vi "Generate Header Vectors.vi"(0 "RFFE RegRead Command in":refnum<class "RFFE RegRead Command.lvclass">, 11 "error in (no error)":errorcluster) -> (4 "RFFE RegRead Command out":refnum<class "RFFE RegRead Command.lvclass">, 6 "Header Vectors":string[](array[string]), 15 "error out":errorcluster)   [LabVIEW 2018, in "MIPI RFFE API.lvlib" / "RFFE RegRead Command.lvclass"]
uses:
  RFFE RegRead Command.lvclass
  Standard Command/RFFE Standard Command.lvclass
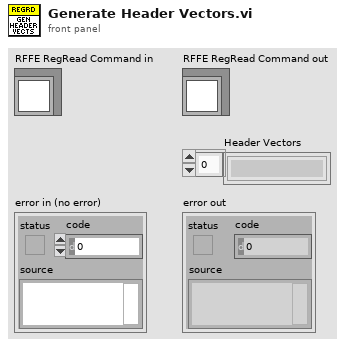
[diagram p1: front panel]
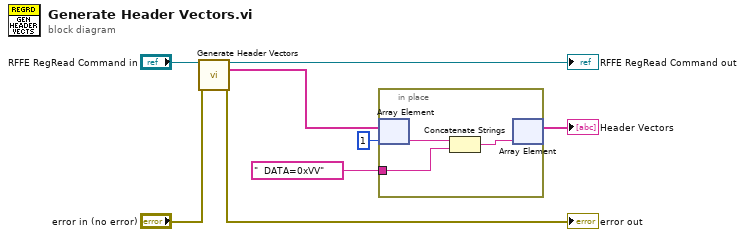
[diagram p0: block diagram]
diagram:
  n1 = call-parent "Generate Header Vectors.vi"("RFFE Command in"="RFFE RegRead Command in", "error in (no error)"="error in (no error)") -> ("RFFE Command out"=→"RFFE RegRead Command out":refnum<class "RFFE RegRead Command.lvclass">, "Header Vectors"=w3:string[], "error out"=→"error out":errorcluster)  [unwired: 11 in]
  n2 = in-place {
    in-place-border: "  DATA=0xVV" ("string") -> [w9]
    n3 = in-place-array #1(w3, 1) -> (w11:string)
    n4 = Concatenate Strings(w11, w9) -> (w10:string)
    n5 = in-place-array #1(w10) -> (→"Header Vectors":string[])  [unwired: 1 out]
  }
